vi "On.vi"(0 "reference in":refnum<class "Spindle.lvclass">, 5 "error in (no error)":errorcluster) -> (14 "reference out":refnum<class "Spindle.lvclass">, 19 "error out":errorcluster)   [LabVIEW 2013, in "Spindle.lvclass"]
uses:
  Spindle.lvclass
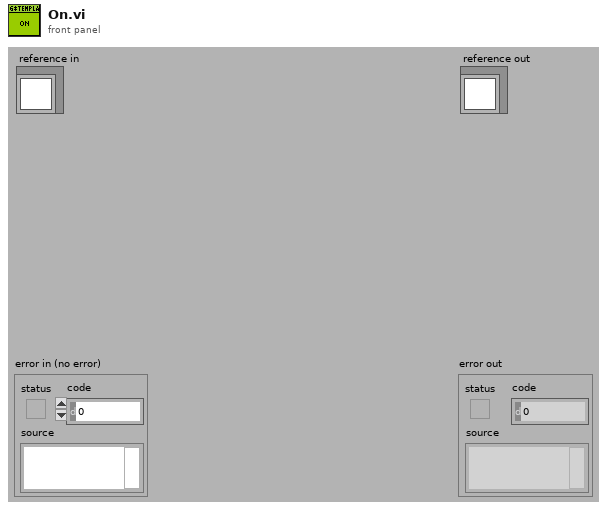
[diagram p1: front panel]
types:
  T1 = typedef "Spindle.lvclass/ObjectAttributes.ctl" = cluster{"Name":string}
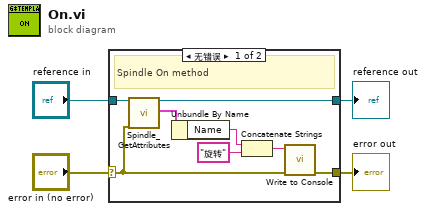
[diagram p0: block diagram]
diagram:
  n1 = case shown="无错误" "error in (no error)" {
    selector: "error in (no error)" -> [w10 w14]
    tunnel: [w12 w14] -> w3
    tunnel: [w9 w13] -> w1
    tunnel: "reference in" -> [w11 w13]
    frame No Error {
      # "Spindle On method"
      n2 = call "Spindle_GetAttributes.vi"("reference in"=w11, "error in (no error)"=w10) -> ("reference out"=w9:refnum<class "Spindle.lvclass">, "attributes"=w8:T1)  [unwired: 14 in, 2 out]
      n3 = Unbundle By Name(w8) -> ("Name"=w7:string)
      n4 = Concatenate Strings(w7, "旋转" ("Input")) -> (w5:string)
      n5 = call "Write to Console.vi"("error in (no error)"=w10, "Input"=w5) -> ("error out"=w12:errorcluster)  [unwired: 9 in]
    }
    frame Error {
    }
  }
  "error out" <- w3
  "reference out" <- w1
